vi "StopOneModule.vi"(8 "error in":errorcluster[](array[cluster]), 11 "Module Name":string) -> (0 "ErrorArray":errorcluster[](array[cluster]))   [LabVIEW 2018]
uses:
  NistPluggableModules/TestClass/Test.lvclass
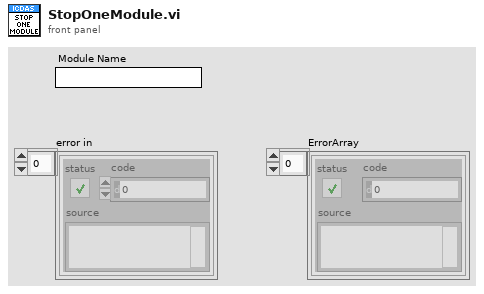
[diagram p1: front panel]
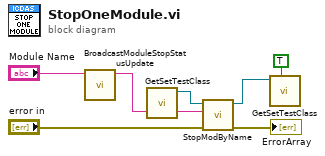
[diagram p0: block diagram]
diagram:
  n1 = call "BroadcastModuleStopStatusUpdate.vi"("Module Name in"="Module Name") -> ("Module Name out"=w1:string)  [unwired: 9 in, 1 out]
  n2 = call "GetSetTestClass.vi"() -> ("Test.lvclass"=w4:refnum<class "Test.lvclass">)  [unwired: 11 in]
  n3 = call "StopModByName.vi"("ErrorArray In"="error in", "Module Name"=w1, "Test.lvclass"=w4) -> ("ErrorArray Out"=→"ErrorArray":errorcluster[], "Test.lvclass"=w5:refnum<class "Test.lvclass">)  [unwired: 4 in, 3 out]
  n4 = call "GetSetTestClass.vi"("Set"=TRUE, "Test.lvclass"=w5) -> ()  [unwired: 9 in, 1 out]
